vi "Get Sender.vi"(8 "error in":errorcluster, 11 "IMessage in":refnum<class "IMessage.lvclass">) -> (0 "error out":errorcluster, 2 "Sender":string, 3 "IMessage out":refnum<class "IMessage.lvclass">)   [LabVIEW 2019, in "IMessage.lvclass"]
uses:
  IMessage.lvclass
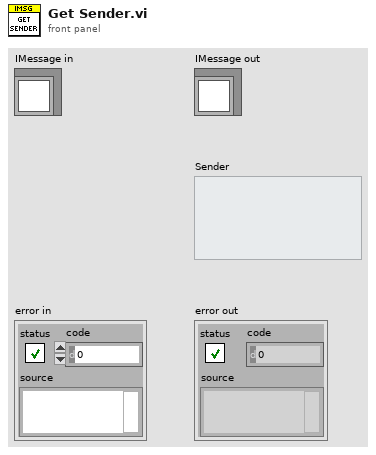
[diagram p1: front panel]
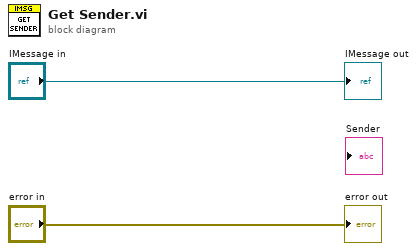
[diagram p0: block diagram]
diagram:
  "error out" <- "error in"
  "IMessage out" <- "IMessage in"
